vi "日期字符串格式至时间格式转换(子VI).vi"(11 "data[0]":string) -> (3 "time stamp":timestamp format="%<%Y/%m/%d %H:%M:%S>T")   [LabVIEW 2016]
uses:
  <vilib>/Utility/miscctls.llb/LVDateTimeRec.ctl
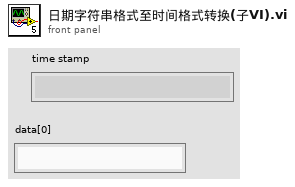
[diagram p1: front panel]
types:
  T1 = typedef "LVDateTimeRec.ctl" = cluster{"fractional second":dbl, "second":i32, "minute":i32, "hour":i32, "day of month":i32, "month":i32, "year":i32, "day of week":i32, "day of year":i32, "DST":i32}
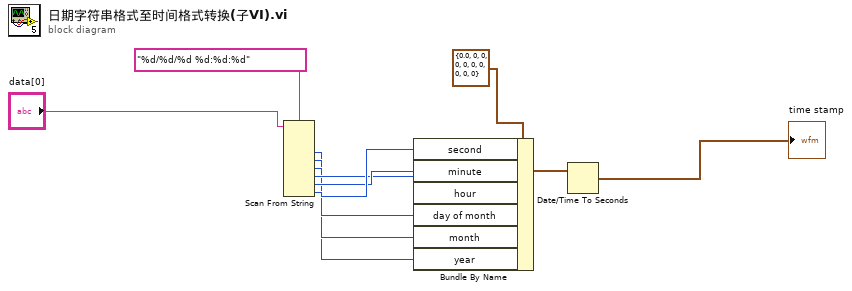
[diagram p0: block diagram]
diagram:
  n1 = Scan From String(format string="%d/%d/%d %d:%d:%d" ("格式字符串"), input string="data[0]") -> (output 1=w4:i32, output 2=w5:i32, output 3=w6:i32, output 4=w7:i32, output 5=w8:i32, output 6=w9:i32)  [unwired: 8 in, 3 out]
  n2 = Bundle By Name(cluster=T1 {"fractional second"=0.0, "second"=0, "minute"=0, "hour"=0, "day of month"=0, "month"=0, "year"=0, "day of week"=0, "day of year"=0, "DST"=0} ("日期时间记录"), "second"=w9, "minute"=w8, "hour"=w7, "day of month"=w6, "month"=w5, "year"=w4) -> (w10:T1)
  n3 = Date/Time To Seconds(2:w10) -> (0:→"time stamp":timestamp)  [unwired: 1 in]
